vi "Periodic Tasks.vi"(8 "error in":errorcluster) -> ()   [LabVIEW 2014]
doc: "This VI runs in parallel to other tasks. It can contain as many user-defined periodic loops as you need. These can carry out PID or other sorts of timed response."
uses:
  Refname/Refname Enum (Actuator).ctl
  <vilib>/Rock Robotics/WPI/RobotDrive/WPI_RobotDriveGetSetRefNum.vi
  lib/Sprocket.lvlib
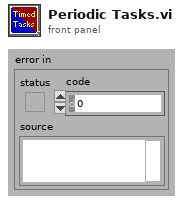
[diagram p1: front panel]
types:
  T1 = typedef "Refname Enum (Actuator).ctl" = enum16{"Drive Motors"}
  T2 = typedef "WPI_RobotDriveDevRef.ctl" = cluster{"DevStatus":errorcluster, "Motors[]":T3[], "Square Inputs":bool, "Max Output":dbl}
  T3 = typedef "WPI_MotorControlDeviceRef.ctl" = cluster{"DeviceStatus":errorcluster, "Type":T4, "PWM":cluster{"Controller":T5, "PWM Channel":T6, "DeadBand":T7}, "CAN":cluster{"Device Number":u8, "Control Mode":T8, "Semaphore":T9, "Max Vout":dbl, "TalonSRX Control Mode":T10}, "Invert":bool, "TransformRef":T11, "InvTransformRef":T11}
  T4 = typedef "WPI_MotorControlType.ctl" = enum16{"PWM", "CAN", "CANTalonSRX"}
  T5 = typedef "FPGA_TypedefDigitalModule.ctl" = enum16{"Controller 1"}
  T6 = typedef "FPGA_DIOPWMChannel.ctl" = enum8{"PWM 0", "PWM 1", "PWM 2", "PWM 3", "PWM 4", "PWM 5", "PWM 6", "PWM 7", "PWM 8", "PWM 9", "PWM MXP 0", "PWM MXP 1", "PWM MXP 2", "PWM MXP 3", "PWM MXP 4", "PWM MXP 5", "PWM MXP 6", "PWM MXP 7", "PWM MXP 8", "PWM MXP 9", "Invalid"}
  T7 = typedef "WPI_PWMDeadband.ctl" = cluster{"Name":string, "maxPositivePwm":i32, "minPositivePwm":i32, "centerPwm":i32, "maxNegativePwm":i32, "minNegativePwm":i32, "angularRange":u16}
  T8 = typedef "WPI_CANJaguar_ControlMode.ctl" = enum8{"Percent VBus", "Current", "Speed", "Position", "Voltage"}
  T9 = typedef "Semaphore RefNum" = refnum<k1>
  T10 = typedef "WPI_CANTalonSRX_APIControlMode.ctl" = enum8{"Percent VBus", "Speed", "Position", "Slave", "Unchanged / Invalid"}
  T11 = typedef "WPI_PWMTransform_ConPane.ctl" = refnum<vi>
  T12 = typedef "Sprocket.lvlib/Action.ctl" = cluster{"Name":T13, "Priority":i32, "Data":variant}
  T13 = typedef "Sprocket.lvlib/Action Name.ctl" = enum16{"Drive Left", "Drive Right"}
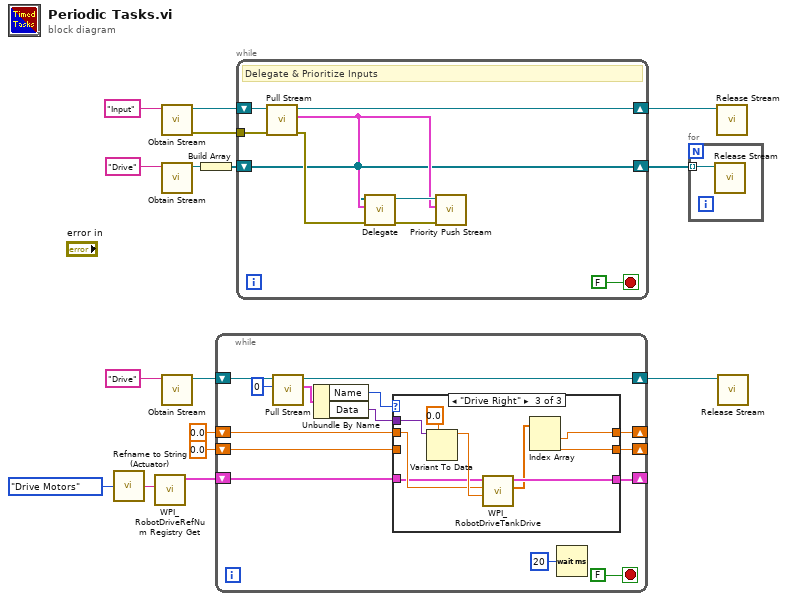
[diagram p0: block diagram]
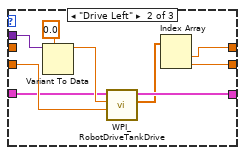
[diagram p3: hidden frame]
diagram:
  n1 = call "Refname to String (Actuator).vi"("Actuator Refname"=Refname_Enum_(Actuator)."Drive Motors") -> ("Refnum Name"=w5:string)
  n2 = call <vilib>:"WPI_RobotDriveRefNum Registry Get.vi"("refnum name"=w5) -> ("RobotDriveDevRef"=w3:T2)  [unwired: 9 in, 1 out]
  n3 = call "Obtain Stream.vi"("Name"="Input") -> ("error out"=w11:errorcluster, "stream out"=w14:refnum<queue>)  [unwired: 9 in]
  n4 = call "Obtain Stream.vi"("Name"="Drive") -> ("stream out"=w13:refnum<queue>)  [unwired: 9 in, 1 out]
  n5 = call "Obtain Stream.vi"("Name"="Drive") -> ("stream out"=w7:refnum<queue>)  [unwired: 9 in, 1 out]
  n6 = Build Array(w13) -> (w12:refnum<queue>[])
  n7 = while {
    shift-right: [w29] -> w6
    shift-left: w7 -> [w30]
    shift-right: [w17] -> _
    shift-left: w3 -> [w22]
    shift-right: [w20] -> _
    shift-left: 0.0 -> [w19]
    shift-right: [w21] -> _
    shift-left: 0.0 -> [w18]
    stop <- FALSE stop-if-true
    n8 = call "Pull Stream.vi"("timeout in ms (-1)"=0, "stream in"=w30) -> ("element"=w25:T12, "queue out"=w29:refnum<queue>)  [unwired: 7 in, 1 out]
    n9 = Unbundle By Name(w25) -> ("Name"=w24:T13, "Data"=w23:variant)
    n10 = case shown="\"Drive Right\"" w24 {
      tunnel: w23 -> [_ w41 w50]
      tunnel: w22 -> [w31 w38 w47]
      tunnel: [w32 w34 w44] -> w21
      tunnel: [w33 w35 w45] -> w20
      tunnel: w19 -> [w33 _ w48]
      tunnel: w18 -> [w32 w39 _]
      tunnel: [w31 w37 w46] -> w17
      frame Default {
      }
      frame "Drive Left" {
        n11 = Variant To Data(type=0.0, Variant=w41) -> (data=w40:dbl)  [unwired: 1 in, 1 out]
        n12 = call <vilib>:"WPI_RobotDriveTankDrive.vi"("Right axis value"=w39, "Left axis value"=w40, "RobotDriveDevRef"=w38) -> ("Motor Values"=w36:dbl[], "RobotDriveDevRef"=w37:T2)  [unwired: 6 in, 1 out]
        n13 = Index Array(array=w36) -> (element #1=w35:dbl, element #2=w34:dbl)  [unwired: 2 in]
      }
      frame "Drive Right" {
        n14 = Variant To Data(type=0.0, Variant=w50) -> (data=w49:dbl)  [unwired: 1 in, 1 out]
        n15 = call <vilib>:"WPI_RobotDriveTankDrive.vi"("Right axis value"=w49, "Left axis value"=w48, "RobotDriveDevRef"=w47) -> ("Motor Values"=w43:dbl[], "RobotDriveDevRef"=w46:T2)  [unwired: 6 in, 1 out]
        n16 = Index Array(array=w43) -> (element #1=w45:dbl, element #2=w44:dbl)  [unwired: 2 in]
      }
    }
    n17 = Wait (ms)(milliseconds to wait=u32 20) -> ()  [unwired: 1 out]
  }
  n18 = while {
    shift-right: [w58] -> w9
    shift-left: w14 -> [w59]
    shift-right: [w52] -> w10
    shift-left: w12 -> [w52]
    tunnel: w11 -> [w54]
    stop <- FALSE stop-if-true
    # "Delegate & Prioritize Inputs"
    n19 = call "Pull Stream.vi"("error in (no error)"=w54, "stream in"=w59) -> ("error out"=w55:errorcluster, "element"=w53:T12, "queue out"=w58:refnum<queue>)  [unwired: 7 in]
    n20 = call "Delegate.vi"("error in (no error)"=w55, "Action"=w53, "Subsystems"=w52) -> ("error out"=w56:errorcluster, "Delegate"=w57:refnum<queue>)  [unwired: 7 in]
    n21 = call "Priority Push Stream.vi"("error in (no error)"=w56, "Action"=w53, "Subsystem in"=w57) -> ()  [unwired: 7 in, 2 out]
  }
  n22 = for {
    tunnel: w10 -> [w61] mode=indexing
    n23 = call "Release Stream.vi"("stream in"=w61) -> ()  [unwired: 9 in, 2 out]
  }
  n24 = call "Release Stream.vi"("stream in"=w9) -> ()  [unwired: 9 in, 2 out]
  n25 = call "Release Stream.vi"("stream in"=w6) -> ()  [unwired: 9 in, 2 out]
